vi "CSM - Destroy Status Change Event.vi"(8 "Error in":errorcluster caption="Error in (no error)", 11 "Status Change Event":refnum<user-event>) -> (0 "Error out":errorcluster)   [LabVIEW 2020, in "Communicable State Machine.lvlib"]
doc: "Release CSM Global Log Event Reference.\n- <b>CSM Global Log Event</b>:\n- <b>Error in</b>: Error cluster\n- <b>Error out</b>: Error cluster\n\n<b>Inputs:</b>\n - <b>Error in</b>:\n - <b>Status Change Event</b>:\n\n<b>Outputs:</b>\n - <b>Error out</b>:"
uses:
  Communicable State Machine.lvlib
  _CSM Status Change Event Data.ctl
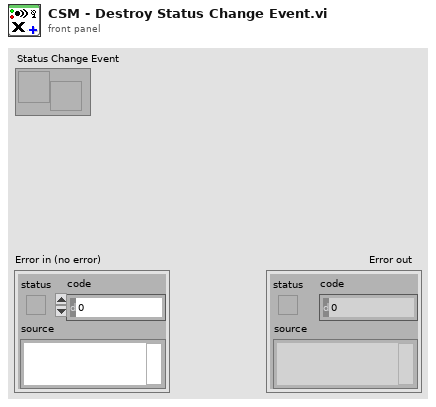
[diagram p1: front panel]
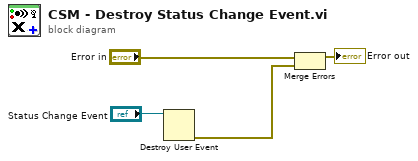
[diagram p0: block diagram]
diagram:
  n1 = Destroy User Event(user event="Status Change Event") -> (error out=w4:errorcluster)  [unwired: 1 in]
  n2 = Merge Errors("Error in", w4) -> (→"Error out":errorcluster)
